vi "ecg_ncs_v6.vi"() -> ()   [LabVIEW 2016]
uses:
  <instrlib>/niUSRP/niUSRP Timestamp.ctl
  C:/Program Files/National Instruments/LabVIEW 2016/examples/Instrument IO/Serial/support/Serial - Settings.ctl
  State.ctl
  <vilib>/Instr/_visa.llb/VISA Configure Serial Port (Instr).vi
  <instrlib>/niUSRP/niUSRP Fetch Rx Data (2D CDB).vi
  <instrlib>/niUSRP/niUSRP Write Tx Data (2D CDB).vi
panel:
  in  "maxWrite":i32=2000
  out "size(s) 2":i32
  out "size(s)":i32
  in  "File Name 2":string="Test"
  in  "Path 2":path=path "D:/Research/SummerFall17Spring18/CnC/NCS/EcgNcsCorrelation/Labview Codes/ECG_NCS"
  out "#Loop = #Packets Received":i32
  out "ECGsample":i16
  out "PhNcs":dbl[](array[numeric])
  out "AmpNcs":dbl[](array[numeric])
  out "AmpNcsDS":dbl[](array[numeric])
  out "PhNcsDS":dbl[](array[numeric])
  out "error IO 2":errorcluster={"status"=FALSE, "code"=-1074118647, "source"=""}
  in  "Serial Settings":T1={"baud rate"=57600, "data bits"=8, "parity"=enum."None", "stop bits"=10, "flow control"=0} {"flow control" items=["None"=0, "XON/XOFF"=1, "RTS/CTS"=2, "DTR/DSR"=4]; "stop bits" items=["1.0"=10, "1.5"=15, "2.0"=20]; "data bits" min=5 max=8 step=1; "baud rate" items=["75"=75, "110"=110, "134"=134, "150"=150, "300"=300, "600"=600, "1200"=1200, "1800"=1800, "2400"=2400, "4800"=4800, "7200"=7200, "9600"=9600, "14400"=14400, "19200"=19200, "28800"=28800, "38400"=38400, "56000"=56000, "57600"=57600, "115200"=115200, "128000"=128000, "230400"=230400]}
  in  "VISA resource name":refnum<visa-resource-name>="bmd101"
  out "ECG":i16(graph)
  in  "byte count":u32=1
  out "Coerced Rx IQ Rate":dbl
  in  "Sampling Rate":i32=500
  out "Gain":dbl=-15.0
  out "Bandwidth":dbl=56000000.0
  out "Coerced Carrier Frequency":dbl=2000000000.0 format="%#.17g"
  out "Coerced Tx IQ rate":dbl=1000000.0
  out "error IO":errorcluster={"status"=FALSE, "code"=-1074118647, "source"=""}
  in  "Rx Number of Samples":i32=6000
  in  "Tab Control 2":enum32{"NI-294x/295x", "NI-2900/2901"}(tab)=enum."NI-2900/2901"
  in  "Rx carrier frequency [Hz]":dbl=2000000000.0 format="%#_6p"
  in  "Tx carrier frequency [Hz]":dbl=1000000000.0 format="%#_6p"
  in  "Start Trigger Time":T2={"whole seconds"=1, "fractional seconds"=0.0}
  in  "Tab Control":T3(tab)
  out "NCS tag Amp":dbl[](graph)=[0.011967714738528729, 0.012021355192189592, 0.012015275039596582, 0.011969166030167903, 0.011958890166168242, 0.012007893820858737, 0.012022893722444085, 0.011978222225113794, 0.011969989939463181, 0.012003099640895068]
  out "NCS tag Phase":dbl[](graph)=[0.011967714738528729, 0.012021355192189592, 0.012015275039596582, 0.011969166030167903, 0.011958890166168242, 0.012007893820858737, 0.012022893722444085, 0.011978222225113794, 0.011969989939463181, 0.012003099640895068]
  out "Tag Amp":dbl[](graph)
  out "Tag Phase":dbl[](graph)
  out "Tx Waveform Graph":waveform(dbl)[](graph)
  in  "Stop":bool
  in  "Tone Amplitude":dbl=0.707 step=0.05 format="%#.6g"
  in  "Tone  Frequency":dbl=5000.0 format="%#_6p"
  in  "Tx Waveform Size":dbl=2000.0
  in  "Device Name":refnum<k15>="MyB200"
  in  "Tx Gain":dbl=28.0 format="%#_6f"
  in  "Tx IQ Rate":dbl=1000000.0 format="%#_6p"
  in  "Rx Gain":dbl=32.0 format="%#_6f"
  in  "Rx IQ Rate":dbl=1000000.0 format="%#_6p"
  # "Rx Settings"
  # "Tx Settings"
  # "Note that on the NI-2900 and NI-2901, both Rx channels share an LO and both Tx channels share an LO. However, on the NI-294x/295x devices, Rx and Tx of channel 0 share an LO and Rx and Tx of channel 1 share an LO."
  # "Rx: Number of samples should be 1e6/512 in one loop."
  # "This Tx graph should always have end and start tied up since this is being sent in a loop continuously. Otherwise phase jumps will be noticed."
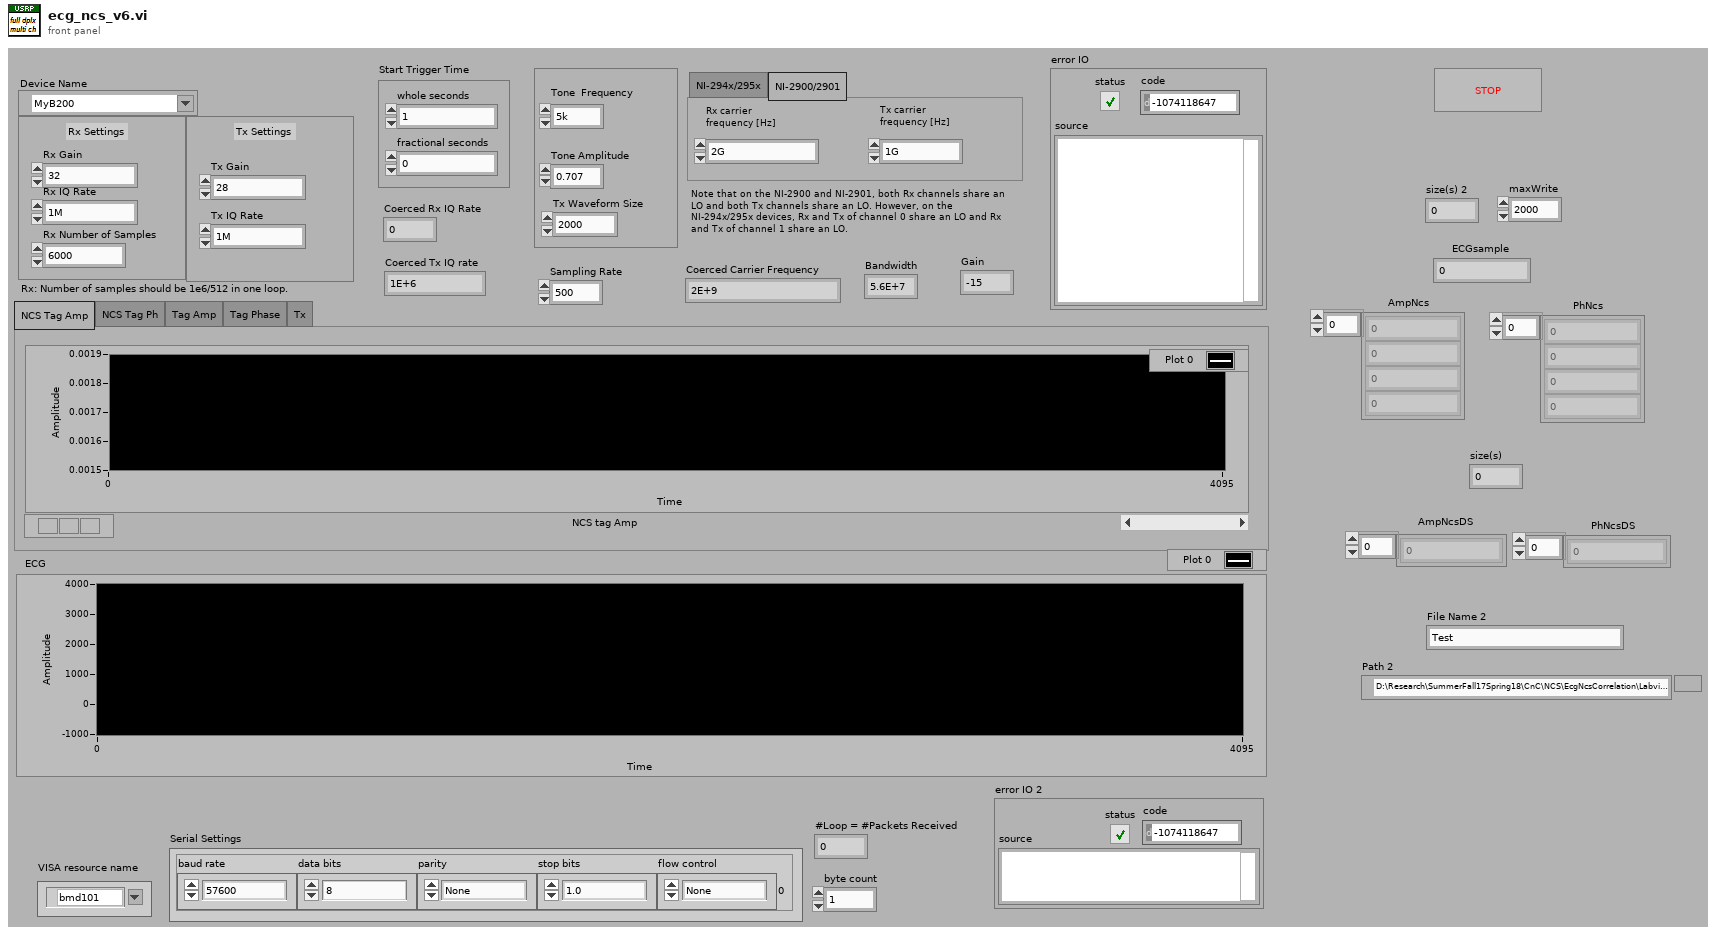
[diagram p1: front panel]
types:
  T1 = typedef "Serial - Settings.ctl" = cluster{"baud rate":u32, "data bits":u16, "parity":enum16{"None", "Odd", "Even", "Mark", "Space"}, "stop bits":u16, "flow control":u16}
  T2 = typedef "niUSRP Timestamp.ctl" = cluster{"whole seconds":u64, "fractional seconds":dbl}
  T3 = enum32{"NCS Tag Amp", "NCS Tag Ph", "Tag Amp", "Tag Phase", "Tx"}
  T4 = typedef "State.ctl" = enum16{"Initialize", "get byte", "check", "packet received", "packet approved"}
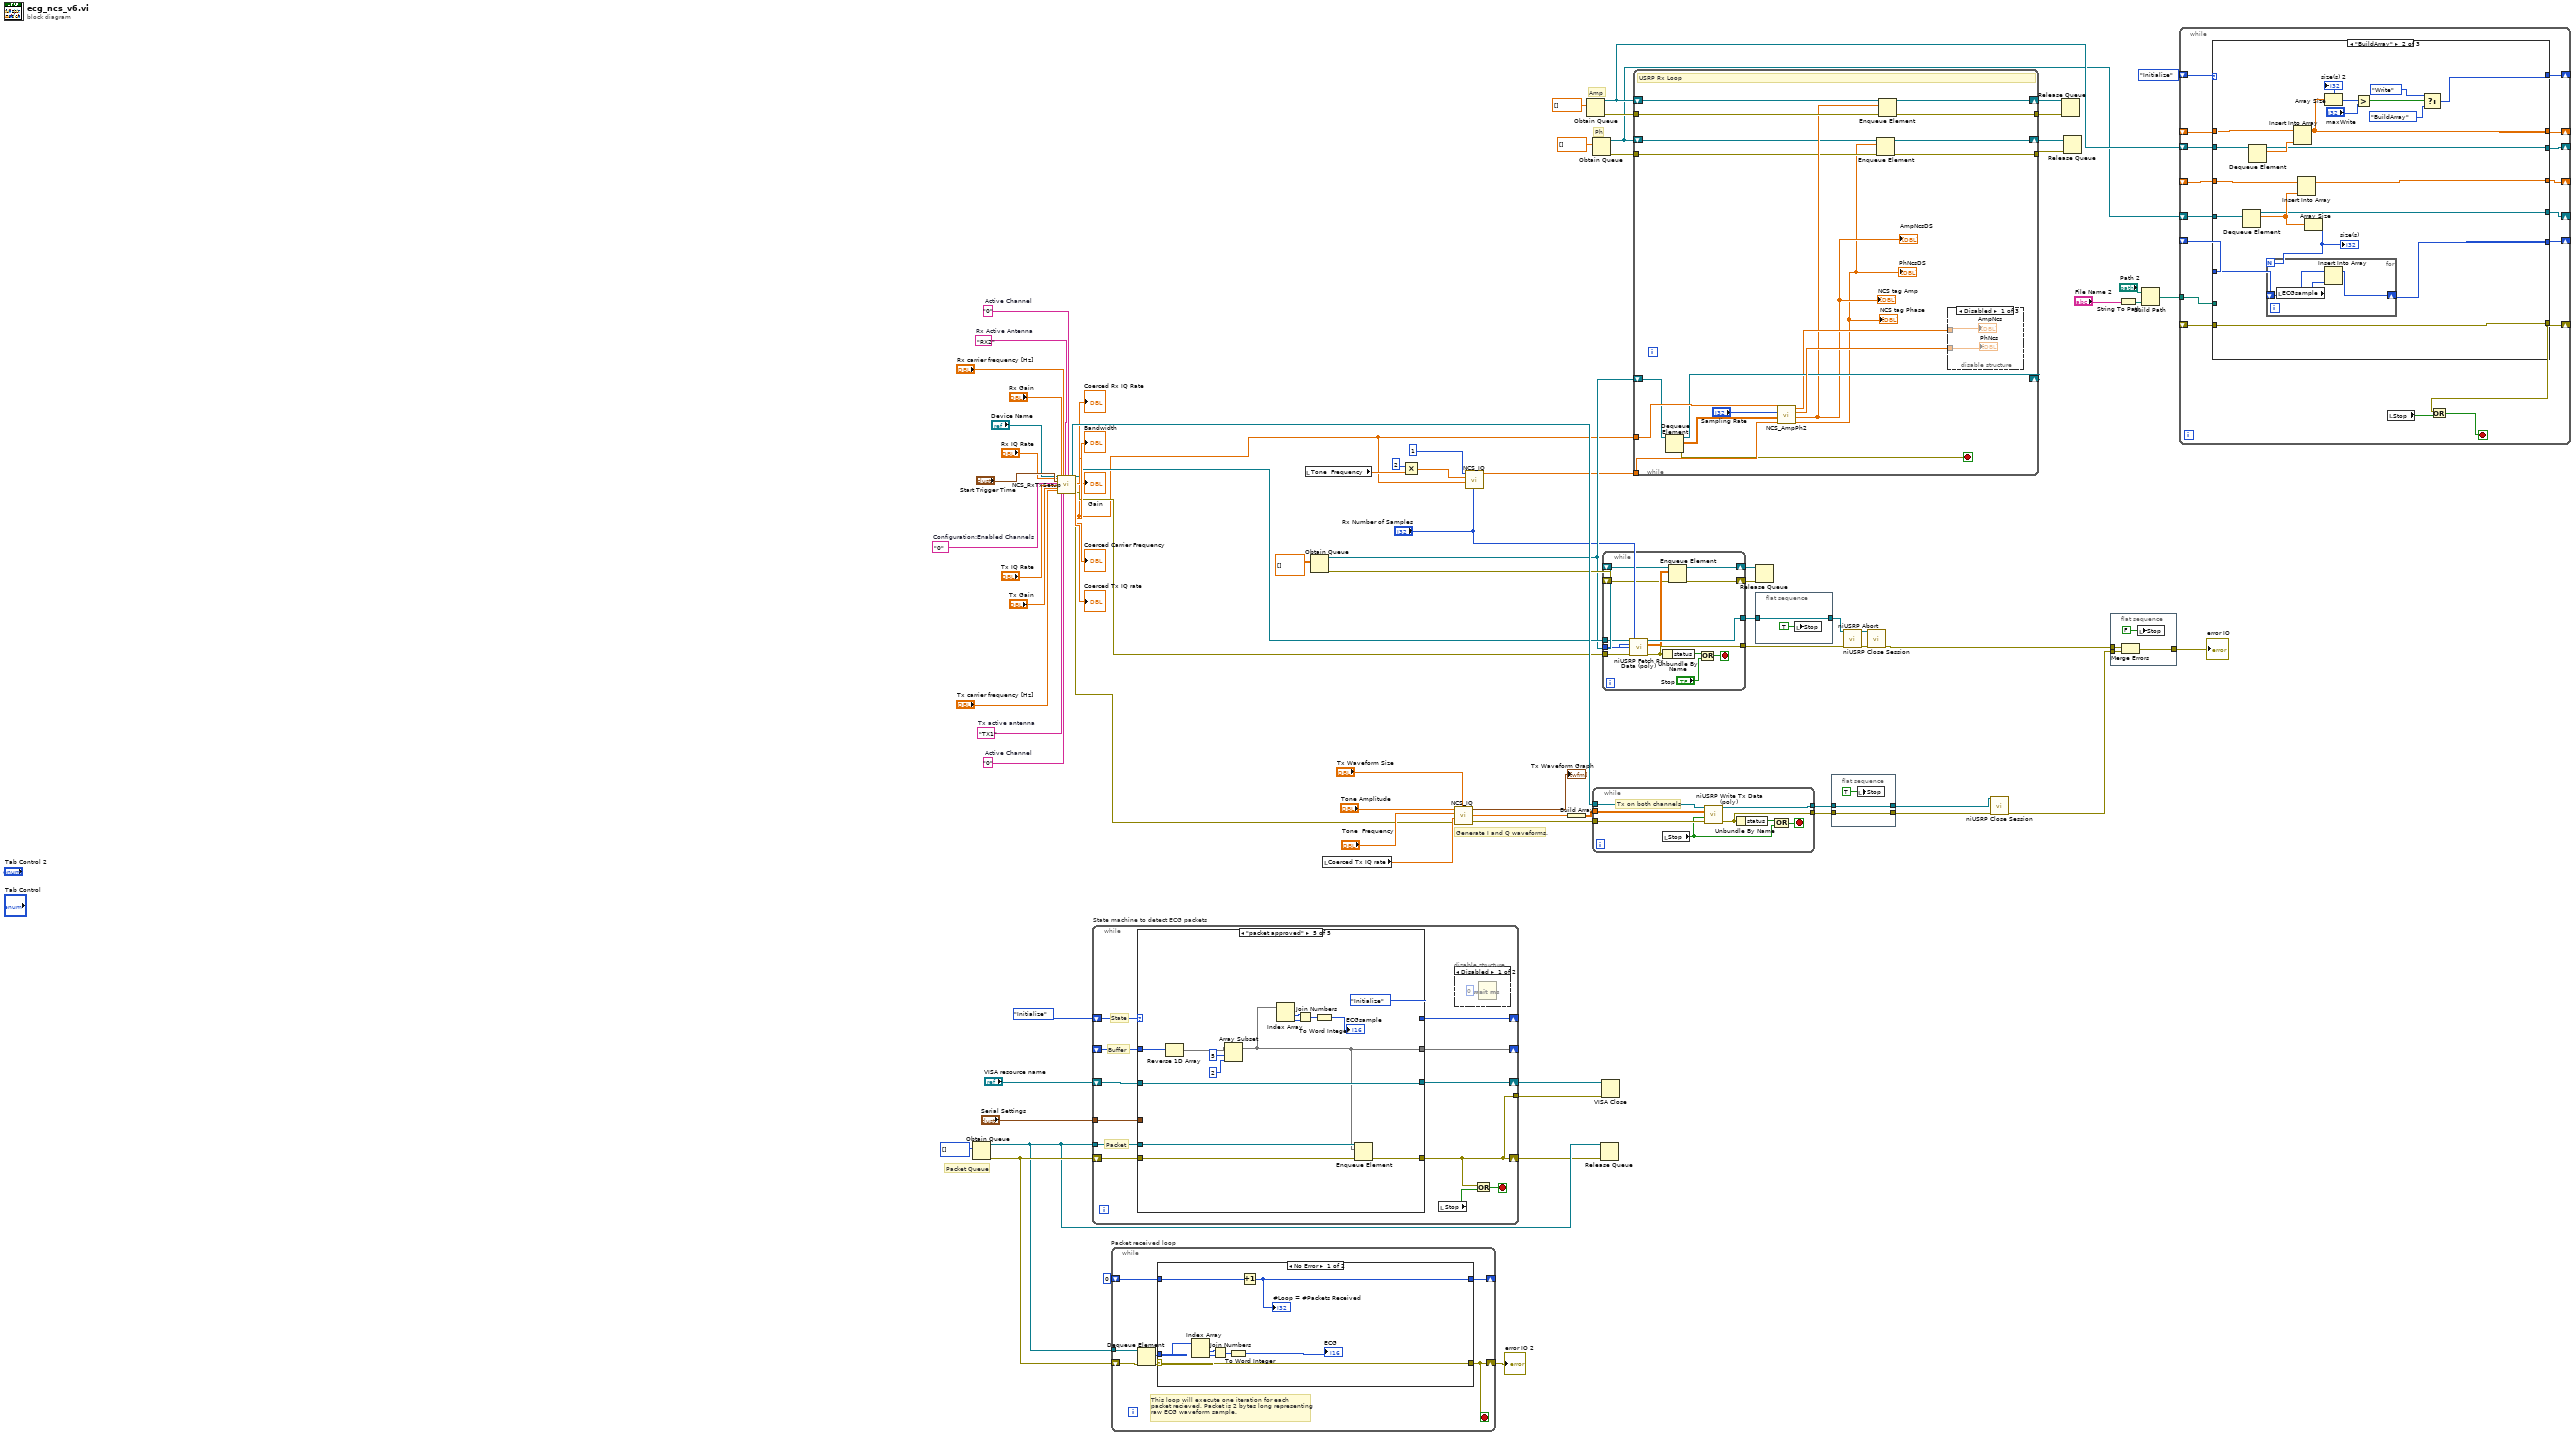
[diagram p0: block diagram]
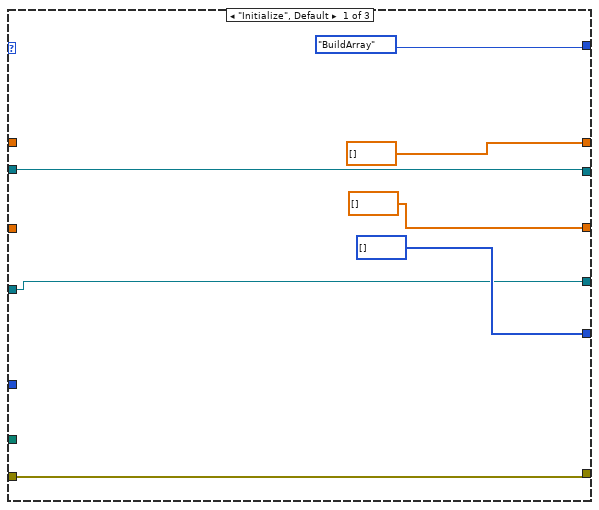
[diagram p2: hidden frame]
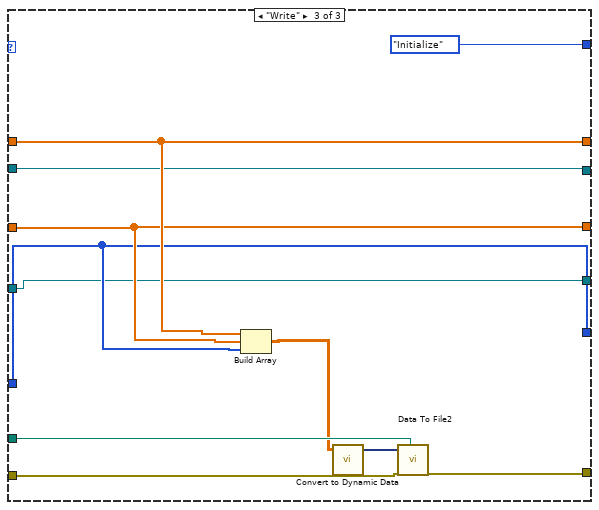
[diagram p3: hidden frame]
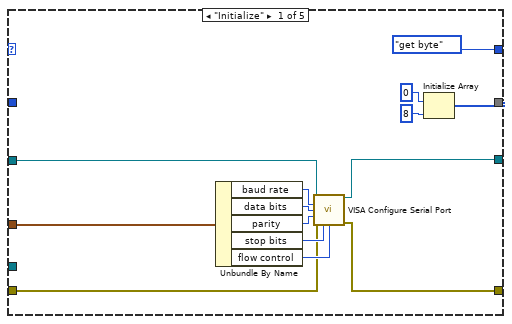
[diagram p6: hidden frame]
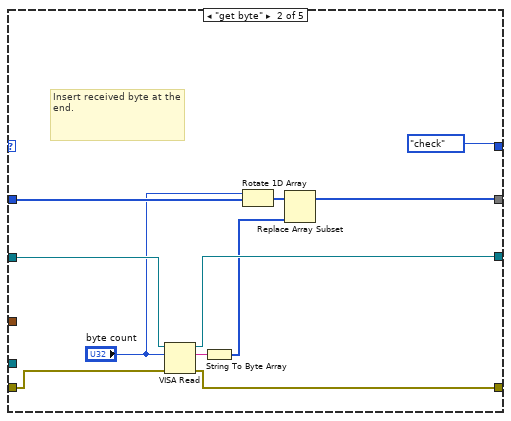
[diagram p7: hidden frame]
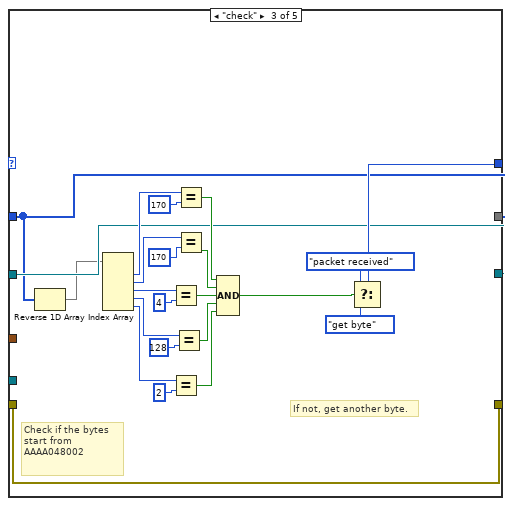
[diagram p8: hidden frame]
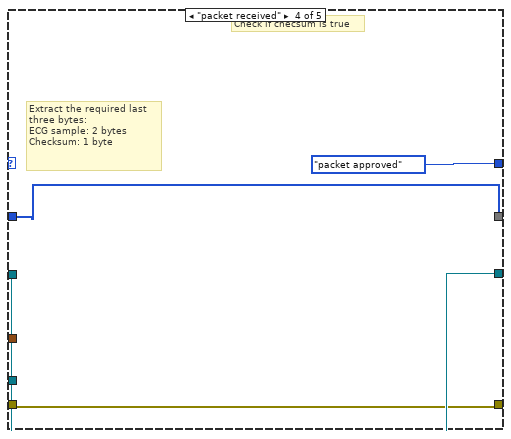
[diagram p9: hidden frame]
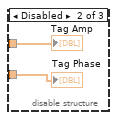
[diagram p10: hidden frame]
diagram:
  w41 = "0"  # Active Channel
  w42 = "0"  # Active Channel
  w71 = "RX2"  # Rx Active Antenna
  w67 = "TX1"  # Tx active antenna
  w56 = "0"  # Configuration:Enabled Channels
  # "Ph"
  # "Amp"
  # "Packet Queue"
  # "Generate I and Q waveforms."
  n1 = Obtain Queue(element data type=u8[] []) -> (queue out=w37:refnum<queue>, error out=w38:errorcluster)  [unwired: 4 in, 1 out]
  n2 = call "NCS_RxTxSetup.vi"("IVI Refnum in"="Device Name", "Rx IQ Rate"="Rx IQ Rate", "Start Trigger Time"="Start Trigger Time", "Configuration:Enabled Channels"=w56, "Tx IQ Rate"="Tx IQ Rate", "Tx Gain"="Tx Gain", "Tx carrier frequency [Hz]"="Tx carrier frequency [Hz]", "Rx Gain"="Rx Gain", "Tx active antenna"=w67, "Rx carrier frequency [Hz]"="Rx carrier frequency [Hz]", "Active Channel"=w41, "Rx Active Antenna"=w71, "Active Channel 2"=w42) -> ("session handle out"=w78:refnum<k15>, "IVI Refnum out"=w27:refnum<k15>, "Coerced Rx IQ Rate"=w17:dbl, "Bandwidth"=→"Bandwidth":dbl, "Gain"=→"Gain":dbl, "Carrier Frequency"=→"Coerced Carrier Frequency":dbl, "IQ Rate 2"=→"Coerced Tx IQ rate":dbl, "error out"=w28:errorcluster)  [unwired: 7 in]
  "Coerced Rx IQ Rate" <- w17
  n3 = while "State machine to detect ECG packets" {
    shift-right: [w81] -> w32
    shift-left: w38 -> [w87]
    shift-right: [w90] -> _
    shift-left: State."Initialize" ("State") -> [w89]
    shift-right: [w86] -> _
    shift-left: _ -> [w88]
    tunnel: w37 -> [w85]
    shift-right: [w84] -> w33
    shift-left: "VISA resource name" -> [w83]
    tunnel: "Serial Settings" -> [w82]
    tunnel: [w81] -> w31
    stop <- w80 stop-if-true
    # "State"
    # "Buffer"
    # "Packet"
    n4 = case shown="\"packet approved\"" w89 {
      tunnel: [w102 w114 w118 w141 w145] -> w86
      tunnel: [State."get byte" ("State") State."check" ("f") w138 State."packet approved" ("State") State."Initialize" ("State")] -> w90
      tunnel: w88 -> [_ w107 w118 w141 w150]
      tunnel: w87 -> [w96 w111 w139 w142 w153]
      tunnel: [w95 w110 w139 w142 w152] -> w81
      tunnel: w85 -> [_ _ _ _ w154]
      tunnel: [w94 w112 w119 w143 w151] -> w84
      tunnel: w83 -> [w93 w113 w119 w143 w151]
      tunnel: w82 -> [w92 _ _ _ _]
      frame "Initialize" {
        n5 = Unbundle By Name(w92) -> ("baud rate"=w101:u32, "data bits"=w100:u16, "parity"=w99:enum16{"None", "Odd", "Even", "Mark", "Space"}, "stop bits"=w98:u16, "flow control"=w97:u16)
        n6 = call-poly "VISA Configure Serial Port"("VISA resource name"=w93, "baud rate (9600)"=w101, "data bits (8)"=w100, "parity (0:none)"=w99, "error in (no error)"=w96, "stop bits (10: 1 bit)"=w98, "flow control (0:none)"=w97) -> ("VISA resource name out"=w94:refnum<visa-resource-name>, "error out"=w95:errorcluster)  [unwired: 3 in, 4 out]
        n7 = Initialize Array(u8 0, 8 ("dimension size")) -> (w102:u8[])
      }
      frame "get byte" {
        # "Insert received byte at the end."
        n8 = VISA Read(VISA resource name=w113, byte count="byte count", error in (no error)=w111) -> (VISA resource name out=w112:refnum<visa-resource-name>, read buffer=w109:string, error out=w110:errorcluster)  [unwired: 1 out]
        n9 = String To Byte Array(string=w109) -> (unsigned byte array=w108:u8[])
        n10 = Rotate 1D Array(1:w107, 2:"byte count") -> (0:w115:u8[])
        n11 = Replace Array Subset(array=w115, new element=w108) -> (w114:u8[])  [unwired: 1 in]
      }
      frame "check" {
        # "If not, get another byte."
        # "Check if the bytes start from AAAA048002"
        n12 = Reverse 1D Array(array=w118) -> (reversed array=w117:u8[])
        n13 = Index Array(array=w117) -> (element #1=w125:u8, element #2=w124:u8, element #3=w123:u8, element #4=w122:u8, element #5=w121:u8)  [unwired: 5 in]
        n14 = Equal?(x=w123, y=u8 4 ("element")) -> (x = y?=w128:bool)
        n15 = Equal?(x=w121, y=u8 2 ("element")) -> (x = y?=w126:bool)
        n16 = Equal?(x=w122, y=u8 128 ("element")) -> (x = y?=w127:bool)
        n17 = Equal?(x=w125, y=u8 170 ("element")) -> (x = y?=w130:bool)
        n18 = Equal?(x=w124, y=u8 170 ("element")) -> (x = y?=w129:bool)
        n19 = Compound Arithmetic op=AND(w130, w129, w128, w127, w126) -> (w120:bool)
        n20 = Select(t=State."packet received" ("f"), s=w120, f=State."get byte") -> (s? t:f=w138:T4)
      }
      frame "packet received" {
        # "Check if checsum is true"
        # "Extract the required last three bytes: \nECG sample: 2 bytes\nChecksum: 1 byte"
      }
      frame "packet approved" {
        n21 = Reverse 1D Array(array=w150) -> (reversed array=w149:u8[])
        n22 = Array Subset(array=w149, index=5, length=2 ("index")) -> (w145:u8[])
        n23 = Index Array(array=w145) -> (element #1=w148:u8, element #2=w147:u8)  [unwired: 2 in]
        n24 = Join Numbers(hi=w148, lo=w147) -> ((hi.lo)=w146:u16)
        n25 = To Word Integer(number=w146) -> (16bit integer=→"ECGsample":i16)
        n26 = Enqueue Element(queue=w154, element=w145, error in (no error)=w153) -> (error out=w152:errorcluster)  [unwired: 1 in, 2 out]
      }
    }
    n27 = local read "Stop"() -> (w79:bool)
    n28 = disable-structure shown="Disabled" {
      frame Disabled {
        n29 = Wait (ms)(milliseconds to wait=u32 0) -> ()  [unwired: 1 out]
      }
      frame Enabled {
      }
    }
    n30 = Or(x=w81, y=w79) -> (x .or. y?=w80:bool)
  }
  n31 = while "Packet received loop" {
    shift-right: [w160] -> w34
    shift-left: w38 -> [w164]
    tunnel: w37 -> [w163]
    shift-right: [w158] -> _
    shift-left: 0 -> [w159]
    stop <- w160 stop-if-true
    # "This loop will execute one iteration for each\npacket recieved. Packet is 2 bytes long representing \nraw ECG waveform sample."
    n32 = Dequeue Element(queue=w163, error in (no error)=w164) -> (element=w162:u8[], error out=w161:errorcluster)  [unwired: 1 in, 2 out]
    n33 = case shown="No Error" w161 {
      selector: w161 -> [w166 w174]
      tunnel: w162 -> [w172 _]
      tunnel: [w166 w174] -> w160
      tunnel: w159 -> [w168 w173]
      tunnel: [w167 w173] -> w158
      frame No Error {
        n34 = Index Array(array=w172) -> (element #1=w171:u8, element #2=w170:u8)  [unwired: 2 in]
        n35 = Join Numbers(hi=w171, lo=w170) -> ((hi.lo)=w169:u16)
        n36 = To Word Integer(number=w169) -> (16bit integer=→"ECG":i16)
        n37 = Increment(x=w168) -> (x+1=w167:i32)
        "#Loop = #Packets Received" <- w167
      }
      frame Error {
      }
    }
  }
  "error IO 2" <- w34
  n38 = local read "Tone  Frequency"() -> (w55:dbl)
  n39 = Obtain Queue(element data type=dbl[][] []) -> (queue out=w21:refnum<queue>, error out=w24:errorcluster)  [unwired: 4 in, 1 out]
  n40 = local read "Coerced Tx IQ rate"() -> (w51:dbl)
  n41 = Multiply(x=2, y=w55) -> (x*y=w18:dbl)
  n42 = call "NCS_IQ.vi"("Tone Amplitude"="Tone Amplitude", "Waveform Size"="Tx Waveform Size", "Tone Frequency"="Tone  Frequency", "Coerced IQ rate"=w51, "error in (no error)"=w28) -> ("IQ waveform"=→"Tx Waveform Graph":waveform(dbl)[], "IQ waveform array"=w49:cdb[], "error out"=w50:errorcluster)  [unwired: 1 in]
  n43 = call "NCS_IQ.vi"("Tone Amplitude"=1, "Waveform Size"="Rx Number of Samples", "Tone Frequency"=w18, "Coerced IQ rate"=w17) -> ("IQ waveform array"=w20:cdb[])  [unwired: 2 in, 2 out]
  n44 = Build Array(w49) -> (w75:cdb[][])
  n45 = Obtain Queue(element data type=dbl[] []) -> (queue out=w2:refnum<queue>, error out=w9:errorcluster)  [unwired: 4 in, 1 out]
  n46 = Obtain Queue(element data type=dbl[] []) -> (queue out=w1:refnum<queue>, error out=w3:errorcluster)  [unwired: 4 in, 1 out]
  n47 = while {
    tunnel: w78 -> [w182]
    tunnel: w50 -> [w181]
    tunnel: [w179] -> w66
    tunnel: [w177] -> w62
    tunnel: w75 -> [w175]
    stop <- w178 stop-if-true
    # "Tx on both channels"
    n48 = local read "Stop"() -> (w176:bool)
    n49 = call-poly <instrlib>:"niUSRP Write Tx Data (poly).vi"("session handle"=w182, "data"=w175, "end of data?"=w176, "error in (no error)"=w181) -> ("session handle out"=w177:refnum<k15>, "error out"=w179:errorcluster)  [unwired: 10 in]
    n50 = Unbundle By Name(w179) -> ("status"=w180:bool)
    n51 = Compound Arithmetic op=OR(w180, w176) -> (w178:bool)
  }
  n52 = Release Queue(queue=w37, error in (no error)=w32) -> ()  [unwired: 1 in, 3 out]
  n53 = VISA Close(VISA resource name=w33, error in (no error)=w31) -> ()  [unwired: 1 out]
  n54 = while {
    tunnel: w28 -> [w195]
    tunnel: w27 -> [w194]
    tunnel: [w193] -> w26
    tunnel: [w185] -> w25
    shift-right: [w189] -> w23
    shift-left: w24 -> [w190]
    shift-right: [w188] -> w22
    shift-left: w21 -> [w192]
    tunnel: "Rx Number of Samples" -> [w187]
    stop <- w184 stop-if-true
    n55 = call-poly <instrlib>:"niUSRP Fetch Rx Data (poly).vi"("session handle"=w194, "number of samples"=w187, "error in (no error)"=w195) -> ("session handle out"=w193:refnum<k15>, "data"=w191:cdb[][], "error out"=w185:errorcluster)  [unwired: 9 in, 1 out]
    n56 = Unbundle By Name(w185) -> ("status"=w186:bool)
    n57 = Enqueue Element(queue=w192, element=w191, error in (no error)=w190) -> (queue out=w188:refnum<queue>, error out=w189:errorcluster)  [unwired: 1 in, 1 out]
    n58 = Or(x=w186, y="Stop") -> (x .or. y?=w184:bool)
  }
  n59 = while {
    tunnel: w17 -> [w214]
    shift-right: [w210] -> _
    shift-left: w21 -> [w211]
    tunnel: w20 -> [w208]
    shift-right: [w202] -> w8
    shift-left: w2 -> [w203]
    tunnel: w9 -> [w206]
    tunnel: [w205] -> w7
    shift-right: [w199] -> w5
    shift-left: w1 -> [w200]
    tunnel: [w198] -> w4
    tunnel: w3 -> [w197]
    stop <- w207 stop-if-true
    # "USRP Rx Loop"
    n60 = Dequeue Element(queue=w211) -> (queue out=w210:refnum<queue>, element=w209:dbl[][], error out=w207:errorcluster)  [unwired: 2 in, 1 out]
    n61 = call "NCS_AmpPh2.vi"("IQ"=w208, "data"=w209, "Sampling Rate"="Sampling Rate", "Coerced Rx IQ Rate"=w214) -> ("Phase DownSampled"=w196:dbl[], "Amp DownSampled"=w201:dbl[], "Phase"=w212:dbl[], "Amplitude"=w204:dbl[])  [unwired: 3 in, 1 out]
    "NCS tag Amp" <- w201
    "AmpNcsDS" <- w201
    "NCS tag Phase" <- w196
    "PhNcsDS" <- w196
    n62 = Enqueue Element(queue=w200, element=w196, error in (no error)=w197) -> (queue out=w199:refnum<queue>, error out=w198:errorcluster)  [unwired: 1 in, 1 out]
    n63 = Enqueue Element(queue=w203, element=w201, error in (no error)=w206) -> (queue out=w202:refnum<queue>, error out=w205:errorcluster)  [unwired: 1 in, 1 out]
    n64 = disable-structure shown="Disabled" {
      disable-tunnel: w204 -> [w215 w218 _]
      disable-tunnel: w212 -> [w216 w217 _]
      frame Disabled {
        "AmpNcs" <- w215
        "PhNcs" <- w216
      }
      frame Disabled {
        "Tag Amp" <- w218
        "Tag Phase" <- w217
      }
      frame Enabled {
      }
    }
  }
  n65 = Release Queue(queue=w22, error in (no error)=w23) -> ()  [unwired: 1 in, 3 out]
  n66 = flat-sequence {
    tunnel: [w219] -> w64
    tunnel: w26 -> [w219]
    frame #0 {
      n67 = local write "Stop"(TRUE ("STOP")) -> ()
    }
  }
  n68 = flat-sequence {
    tunnel: [w222] -> w65
    tunnel: w66 -> [w222]
    tunnel: [w221] -> w63
    tunnel: w62 -> [w221]
    frame #0 {
      n69 = local write "Stop"(TRUE ("STOP")) -> ()
    }
  }
  n70 = call <instrlib>:"niUSRP Abort.vi"("session handle"=w64, "error in (no error)"=w25) -> ("session handle out"=w77:refnum<k15>, "error out"=w76:errorcluster)  [unwired: 12 in]
  n71 = call <instrlib>:"niUSRP Close Session.vi"("session handle"=w77, "error in (no error)"=w76) -> ("error out"=w59:errorcluster)  [unwired: 13 in]
  n72 = call <instrlib>:"niUSRP Close Session.vi"("session handle"=w63, "error in (no error)"=w65) -> ("error out"=w61:errorcluster)  [unwired: 13 in]
  n73 = Release Queue(queue=w8, error in (no error)=w7) -> ()  [unwired: 1 in, 3 out]
  n74 = Release Queue(queue=w5, error in (no error)=w4) -> ()  [unwired: 1 in, 3 out]
  n75 = flat-sequence {
    tunnel: w61 -> [w226]
    tunnel: [w225] -> w60
    tunnel: w59 -> [w224]
    frame #0 {
      n76 = Merge Errors(w224, w226) -> (w225:errorcluster)
      n77 = local write "Stop"(FALSE ("STOP")) -> ()
    }
  }
  n78 = String To Path(string="File Name 2") -> (path=w15:path)
  n79 = Build Path(base path="Path 2", name or relative path=w15) -> (appended path=w11:path)
  n80 = while {
    shift-right: [w243] -> _
    shift-left: _ -> [w244]
    shift-right: [w239] -> _
    shift-left: _ -> [w242]
    shift-right: [w240] -> _
    shift-left: _ -> [w241]
    shift-right: [w237] -> _
    shift-left: enum16{"Initialize", "BuildArray", "Write"}."Initialize" -> [w238]
    tunnel: w11 -> [w236]
    shift-right: [w233] -> _
    shift-left: _ -> [w232]
    shift-right: [w230] -> _
    shift-left: w2 -> [w231]
    shift-right: [w228] -> _
    shift-left: w1 -> [w229]
    stop <- w234 stop-if-true
    n81 = case shown="\"BuildArray\"" w238 {
      tunnel: w244 -> [_ w271 w282]
      tunnel: [dbl[] [] w265 w282] -> w243
      tunnel: w242 -> [_ w270 w281]
      tunnel: w241 -> [_ w269 w280]
      tunnel: [i32[] [] w268 w280] -> w240
      tunnel: [dbl[] [] w267 w281] -> w239
      tunnel: [enum16{"Initialize", "BuildArray", "Write"}."BuildArray" w259 enum16{"Initialize", "BuildArray", "Write"}."Initialize"] -> w237
      tunnel: w236 -> [_ _ w283]
      tunnel: [w247 w258 w278] -> w233
      tunnel: w232 -> [w247 w258 w277]
      tunnel: w231 -> [w246 w256 w276]
      tunnel: [w246 w255 w276] -> w230
      tunnel: w229 -> [w245 w254 w275]
      tunnel: [w245 w252 w275] -> w228
      frame "Initialize", Default {
      }
      frame "BuildArray" {
        n82 = Dequeue Element(queue=w254) -> (queue out=w252:refnum<queue>, element=w253:dbl[])  [unwired: 2 in, 2 out]
        n83 = Dequeue Element(queue=w256) -> (queue out=w255:refnum<queue>, element=w257:dbl[])  [unwired: 2 in, 2 out]
        n84 = Insert Into Array(array=w271, new element=w257) -> (w265:dbl[])  [unwired: 1 in]
        n85 = Insert Into Array(array=w270, new element=w253) -> (w267:dbl[])  [unwired: 1 in]
        n86 = Array Size(array=w253) -> (size(s)=w266:i32)
        "size(s)" <- w266
        n87 = for {
          N: w266 -> [_]
          shift-right: [w272] -> w268
          shift-left: w269 -> [w273]
          n88 = local read "ECGsample"() -> (w274:i16)
          n89 = Insert Into Array(array=w273, new element=w274) -> (w272:i32[])  [unwired: 1 in]
        }
        n90 = Array Size(array=w265) -> (size(s)=w264:i32)
        "size(s) 2" <- w264
        n91 = Greater?(x=w264, y="maxWrite") -> (0:w262:bool)
        n92 = Select(t=enum16{"Initialize", "BuildArray", "Write"}."Write", s=w262, f=enum16{"Initialize", "BuildArray", "Write"}."BuildArray") -> (s? t:f=w259:enum16{"Initialize", "BuildArray", "Write"})
      }
      frame "Write" {
        n93 = Build Array(w282, w281, w280) -> (w279:dbl[][])
        n94 = call "Convert to Dynamic Data"("2D Array"=w279) -> ("Dynamic Data Type"=w284:dynamicdata)  [unwired: 3 in]
        n95 = call "Data To File2"("Signals"=w284, "error in (no error)"=w277, "Filename"=w283) -> ("error out"=w278:errorcluster)  [unwired: 14 in, 2 out]
      }
    }
    n96 = local read "Stop"() -> (w235:bool)
    n97 = Or(x=w233, y=w235) -> (x .or. y?=w234:bool)
  }
  "error IO" <- w60
